vi "Table, Get Cell Value, Double.vi"(8 "error in":errorcluster, 9 "col":i32, 10 "row":i32, 11 "Tbl Refnum":refnum<vi>) -> (0 "error out":errorcluster, 2 "cell value":dbl=nan format="%.f", 3 "Tbl Refnum out":refnum<vi>)   [LabVIEW 2010]
doc: "Gets a single table cell double precision floating point value.\nA conversion error will return NaN."
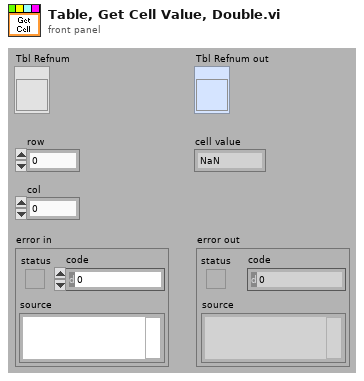
[diagram p1: front panel]
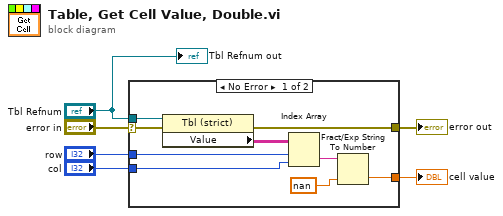
[diagram p0: block diagram]
diagram:
  n1 = case shown="No Error" "error in" {
    selector: "error in" -> [w13 w16]
    tunnel: "Tbl Refnum" -> [w15 _]
    tunnel: [w14 w16] -> w5
    tunnel: "row" -> [w7 _]
    tunnel: "col" -> [w8 _]
    tunnel: [w10 _] -> w1
    frame No Error {
      n2 = property class="Tbl (strict)"(reference=w15, error in=w13) -> (error out=w14:errorcluster, "Value"=w12:string[][])  [unwired: 1 out]
      n3 = Index Array(array=w12, index (row)=w7, index (col)=w8) -> (element=w11:string)
      n4 = Fract/Exp String To Number(string=w11, default (0 dbl)=nan) -> (number=w10:dbl)  [unwired: 2 in, 1 out]
    }
    frame Error {
    }
  }
  "error out" <- w5
  "cell value" <- w1
  "Tbl Refnum out" <- "Tbl Refnum"
